vi "Filter List.get.vi"(11 "selection_dropdown in":refnum<class "selection_dropdown.lvclass">) -> (2 "filter list":string[](array[string]), 3 "selection_dropdown out":refnum<class "selection_dropdown.lvclass">)   [LabVIEW 2024, in "selection_dropdown.lvclass"]
uses:
  selection_dropdown.lvclass
  selection_dropdown.lvclass/selection_dropdown.ctl
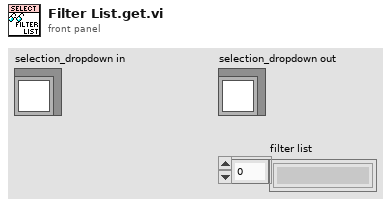
[diagram p1: front panel]
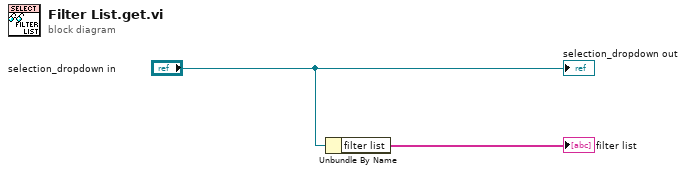
[diagram p0: block diagram]
diagram:
  n1 = Unbundle By Name("selection_dropdown in") -> ("filter list"=→"filter list":string[])
  "selection_dropdown out" <- "selection_dropdown in"
